vi "Grid Visualization Global.vi"() -> ()   [LabVIEW 2020]
panel:
  in  "b 9":dbl
  in  "b 8":dbl
  in  "b 7":dbl
  in  "b 6":dbl
  in  "b 5":dbl
  in  "b 4":dbl
  in  "b 3":dbl
  in  "b 2":dbl=-1.0
  in  "b 1":dbl=-1.0
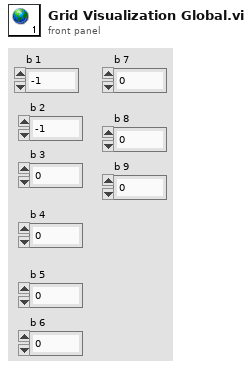
[diagram p1: front panel]
diagram:
